vi "CLD 15 Parsing SubVI.vi"(8 "Fehler (Eingang)":T2, 11 "Alle Zeilen (Eingang)":string[][](array[string])) -> (0 "Fehler (Ausgang)":T2, 3 "Daten (Ausgang)":T1[](array[typedef]))   [LabVIEW 2009]
doc: "CLD 15 - Dieses SubVI wandelt die Array-Daten in das Format um, das in der Spezifikation für CLD 15 vorgegeben ist. Für das Dekodieren der String-Daten gibt es mehrere Möglichkeiten. \n\nIn Case 0 werden feste Positionen für die Zahlen verwendet. In Case 1 werden Text und Zahlen im Daten-String mit Hilfe von regulären Ausdrücke getrennt.\n\nDas Datenformat der Spezifikation wurde als freie Beschriftung kopiert, um die Programmierung zu erleichtern."
uses:
  CLD 15 CSV file data structure.ctl
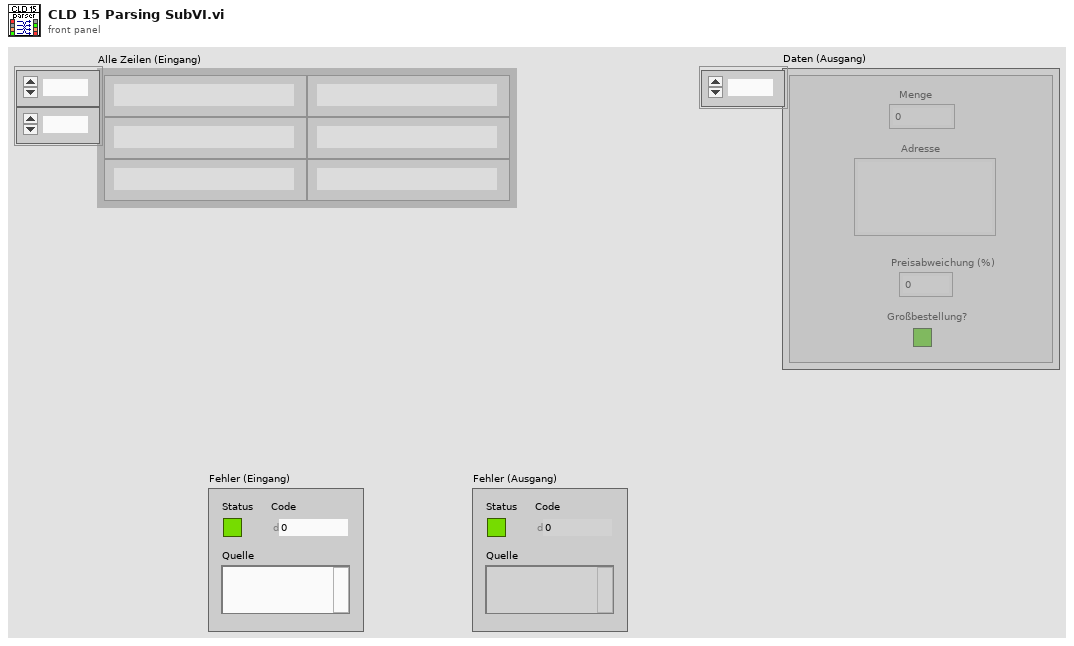
[diagram p1: front panel]
types:
  T1 = typedef "CLD 15 CSV file data structure.ctl" = cluster{"Menge":i32, "Adresse":string, "Preisabweichung (%)":dbl, "Großbestellung?":bool}
  T2 = cluster{"Status":bool, "Code":i32, "Quelle":string}
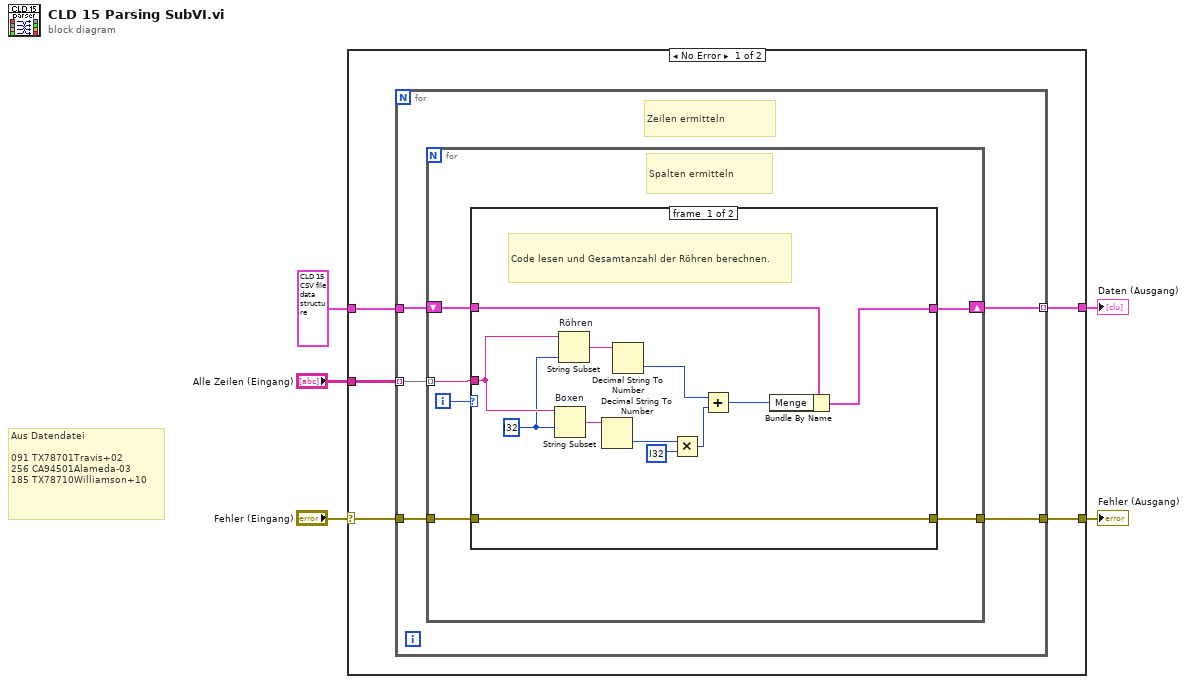
[diagram p0: block diagram]
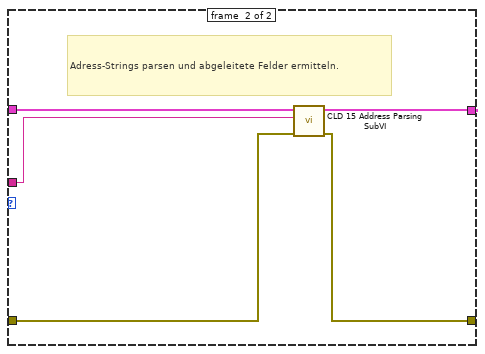
[diagram p2: hidden frame]
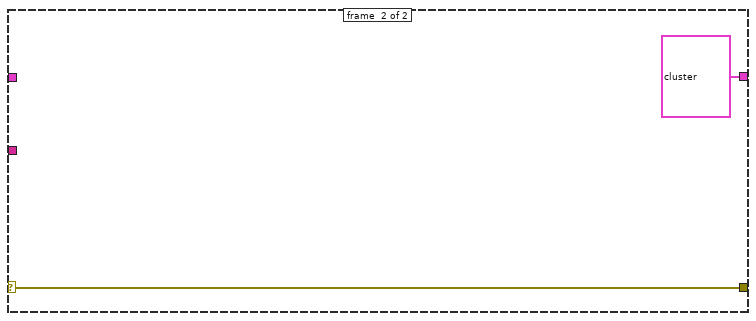
[diagram p3: hidden frame]
diagram:
  # "Aus Datendatei\n\n091\tTX78701Travis+02\n256\tCA94501Alameda-03\n185\tTX78710Williamson+10"
  n1 = case shown="No Error" "Fehler (Eingang)" {
    selector: "Fehler (Eingang)" -> [w7 w39]
    tunnel: [w10 w39] -> w5
    tunnel: T1 ? ("Datenstruktur der CSV-Datei") -> [w9 _]
    tunnel: [w8 T1[] ?] -> w3
    tunnel: "Alle Zeilen (Eingang)" -> [w6 _]
    frame #0 {
      n2 = for {
        tunnel: w7 -> [w15]
        tunnel: [w14] -> w10
        tunnel: w9 -> [w13]
        tunnel: [w12] -> w8 mode=indexing
        tunnel: w6 -> [w11] mode=indexing
        # "Zeilen ermitteln"
        n3 = for {
          tunnel: w15 -> [w18]
          tunnel: [w17] -> w14
          shift-right: [w19] -> w12
          shift-left: w13 -> [w20]
          tunnel: w11 -> [w16] mode=indexing
          i -> [w21]
          # "Spalten ermitteln"
          n4 = case shown="1" w21 {
            tunnel: w16 -> [w33 w38]
            tunnel: w20 -> [w30 w37]
            tunnel: [w29 w36] -> w19
            tunnel: w18 -> [w22 w35]
            tunnel: [w22 w34] -> w17
            frame #0 {
              w23 = i32 ? ("Länge (Rest)")
              # "Code lesen und Gesamtanzahl der Röhren berechnen."
              n5 = String Subset "Boxen"(string=w33, offset (0)=w23) -> (substring=w31:string)  [unwired: 1 in]
              n6 = String Subset "Röhren"(string=w33, length (rest)=w23) -> (substring=w32:string)  [unwired: 1 in]
              n7 = Decimal String To Number(string=w31) -> (number=w27:i32)  [unwired: 2 in, 1 out]
              n8 = Decimal String To Number(string=w32) -> (number=w28:i32)  [unwired: 2 in, 1 out]
              n9 = Multiply(x=w27, y=i32 ?) -> (x*y=w24:i32)
              n10 = Add(x=w28, y=w24) -> (x+y=w25:i32)
              n11 = Bundle By Name(cluster=w30, "Menge"=w25) -> (w29:T1)
            }
            frame #1 {
              # "Adress-Strings parsen und abgeleitete Felder ermitteln."
              n12 = call "CLD 15 Address Parsing SubVI.vi"("Fehler (Eingang)"=w35, "Daten-String (Eingang)"=w38, "Datenstruktur der CSV-Datei (Eingang)"=w37) -> ("Fehler (Ausgang)"=w34:errorcluster, "Datenstruktur der CSV-Datei (Ausgang)"=w36:T1)  [unwired: 7 in]
            }
          }
        }
      }
    }
    frame #1 {
    }
  }
  "Fehler (Ausgang)" <- w5
  "Daten (Ausgang)" <- w3
